vi "登录对话框.vi"() -> (1 "显示文件名":string, 2 "access out":T1)   [LabVIEW 2014]
uses:
  <vilib>/addons/database/Connection.llb/Conn ObjectReference.ctl
  <vilib>/addons/database/NI_Database_API.lvlib
panel:
  in  "Volume of rock sample(cm3)":string
  in  "Sectional area(cm2)":string
  in  "Irreducible water saturation(%)":string
  in  "Outlet pressure(MPa)":string
  in  "Inlet pressure(MPa)":string
  in  "Porosity(%)":string
  in  "Rock sample diameter(cm)":string
  in  "Injection water density(g/cm3)":string
  in  "Simulated oil density(g/cm3)":string
  in  "Air permeability(0.001um2)":string
  in  "Core depth(m)":string
  in  "Pore volume(cm3)":string
  in  "Length of rock sample(cm)":string
  in  "Injection water viscosity(mPa.S)":string
  in  "Simulated oil viscosity(mPa.S)":string
  in  "Experimental temperature(℃)":string
  in  "Lithological character":string
  in  "No.":string
  in  "Date of experiment":timestamp
  in  "Well number":string
  in  "Inspection item":string
  in  "取消按钮":bool
  in  "确定按钮":bool
  in  "Data store path":path
  in  "Document name":string
  # "Store path settings"
  # "Basic data"
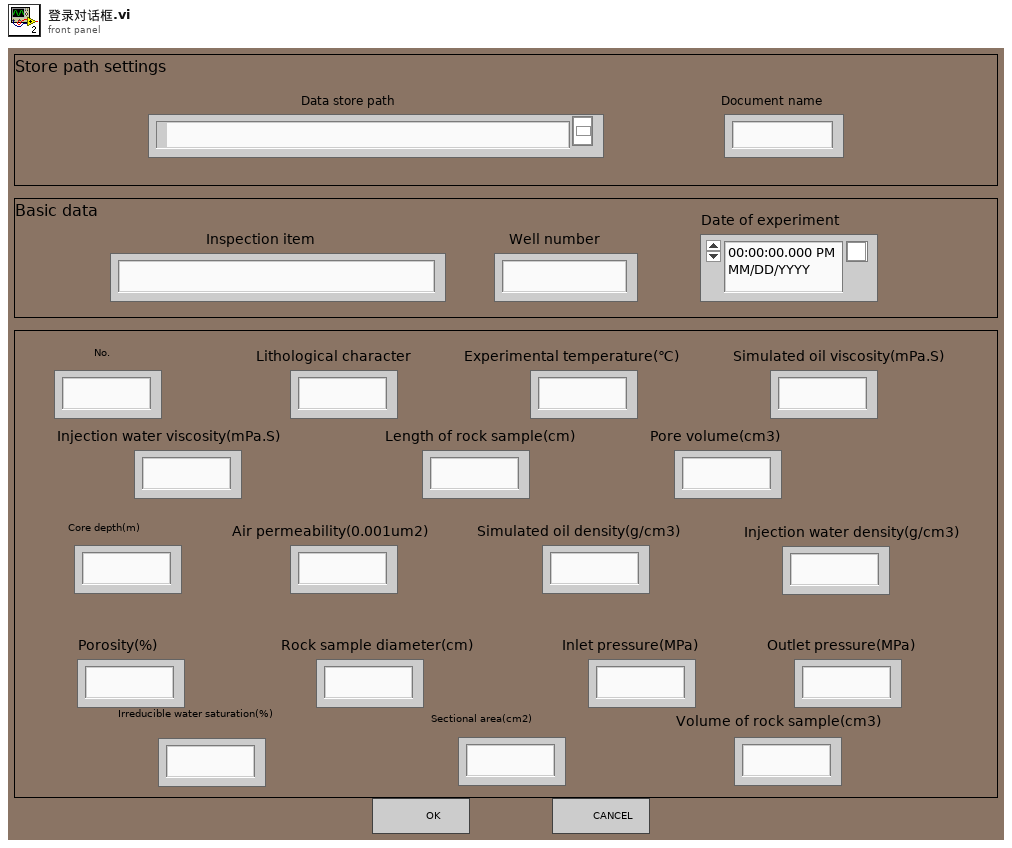
[diagram p1: front panel]
types:
  T1 = typedef "NI_Database_API.lvlib/Conn ObjectReference.ctl" = refnum<k1>
  T2 = cluster{"Inspection item":string, "Well number":string, "date/time string":string, "No.":string, "Lithological character":string, "Experimental temperature(℃)":string, "Simulated oil viscosity(mPa.S)":string, "Injection water viscosity(mPa.S) ":string, "Length of rock sample(cm)":string, "Pore volume(cm3) ":string, "Core depth(m)":string, "Air permeability(0.001um2)":string, "Simulated oil density(g/cm3)":string, "Injection water density(g/cm3)":string, "Porosity(%)":string, "Rock sample diameter(cm)":string, "Inlet pressure(MPa)":string, "Outlet pressure(MPa)":string, "Irreducible water saturation(%)":string, "Sectional area(cm2)":string, "Volume of rock sample(cm3)":string}
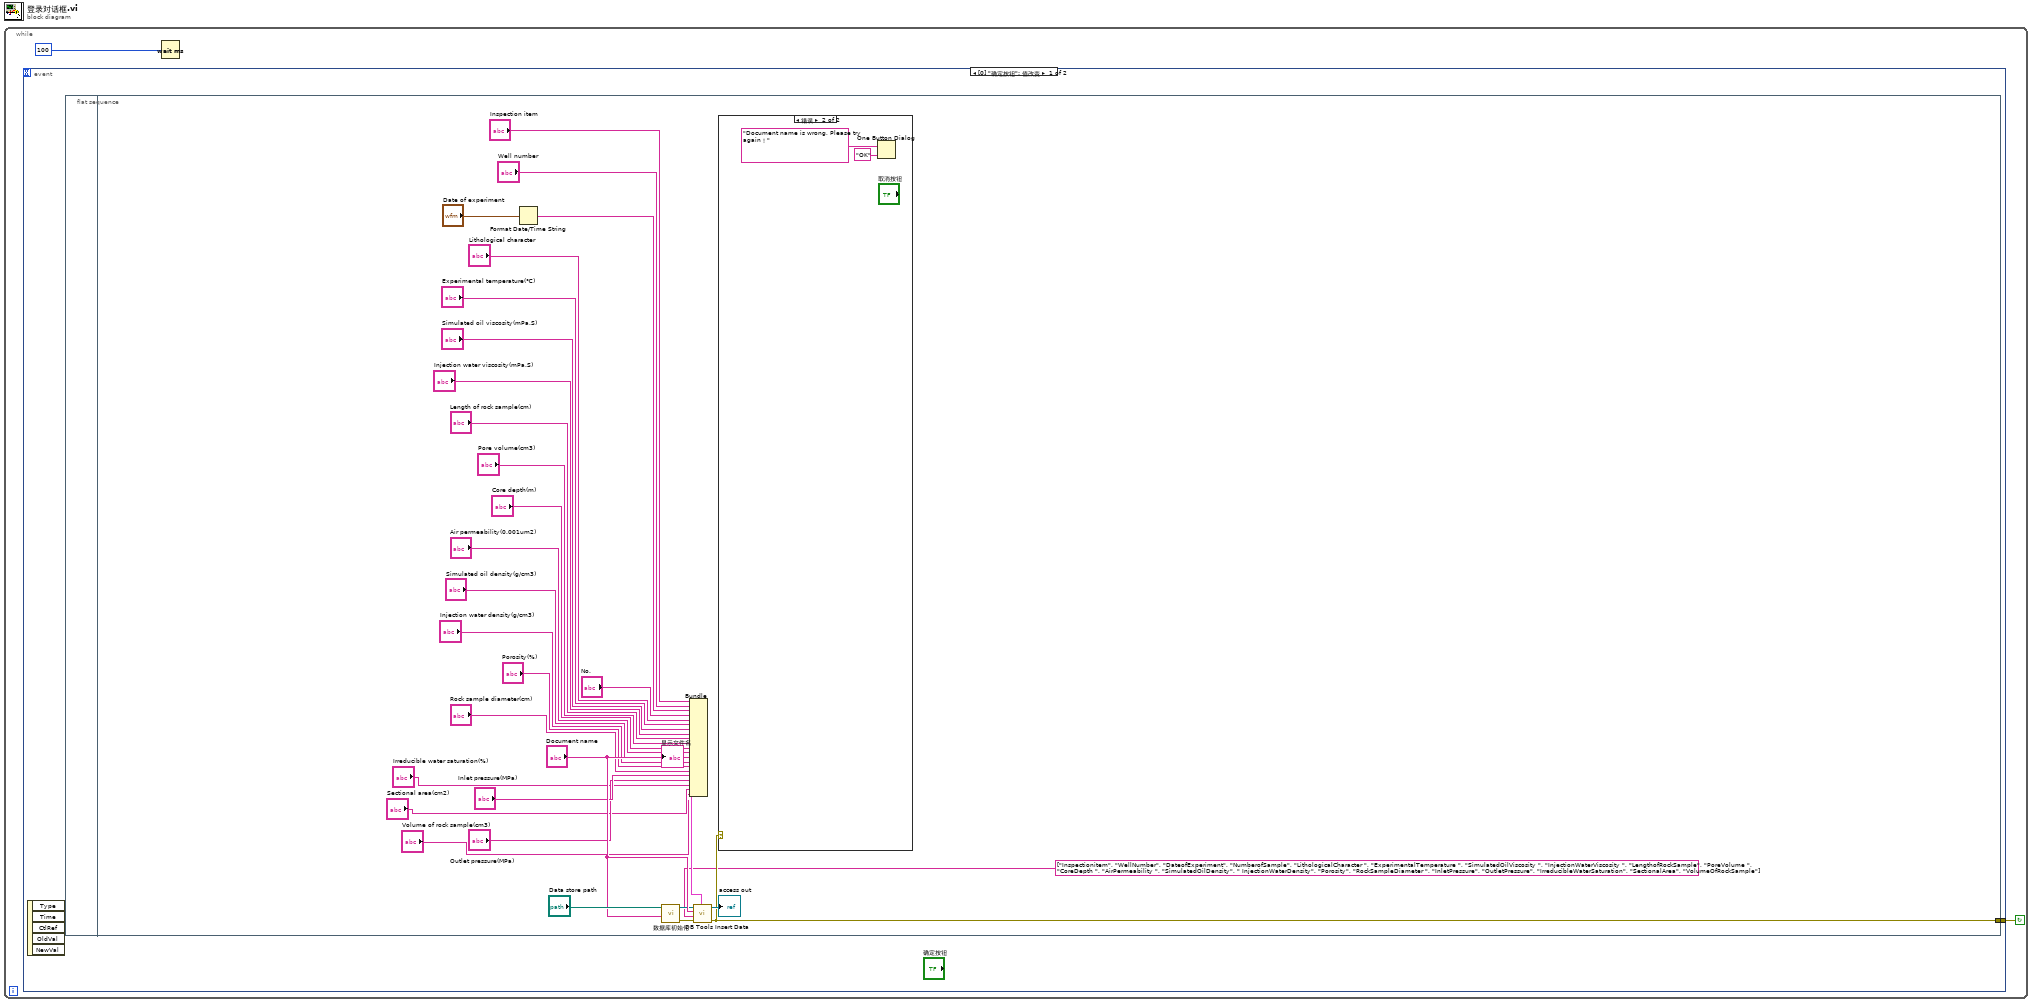
[diagram p0: block diagram]
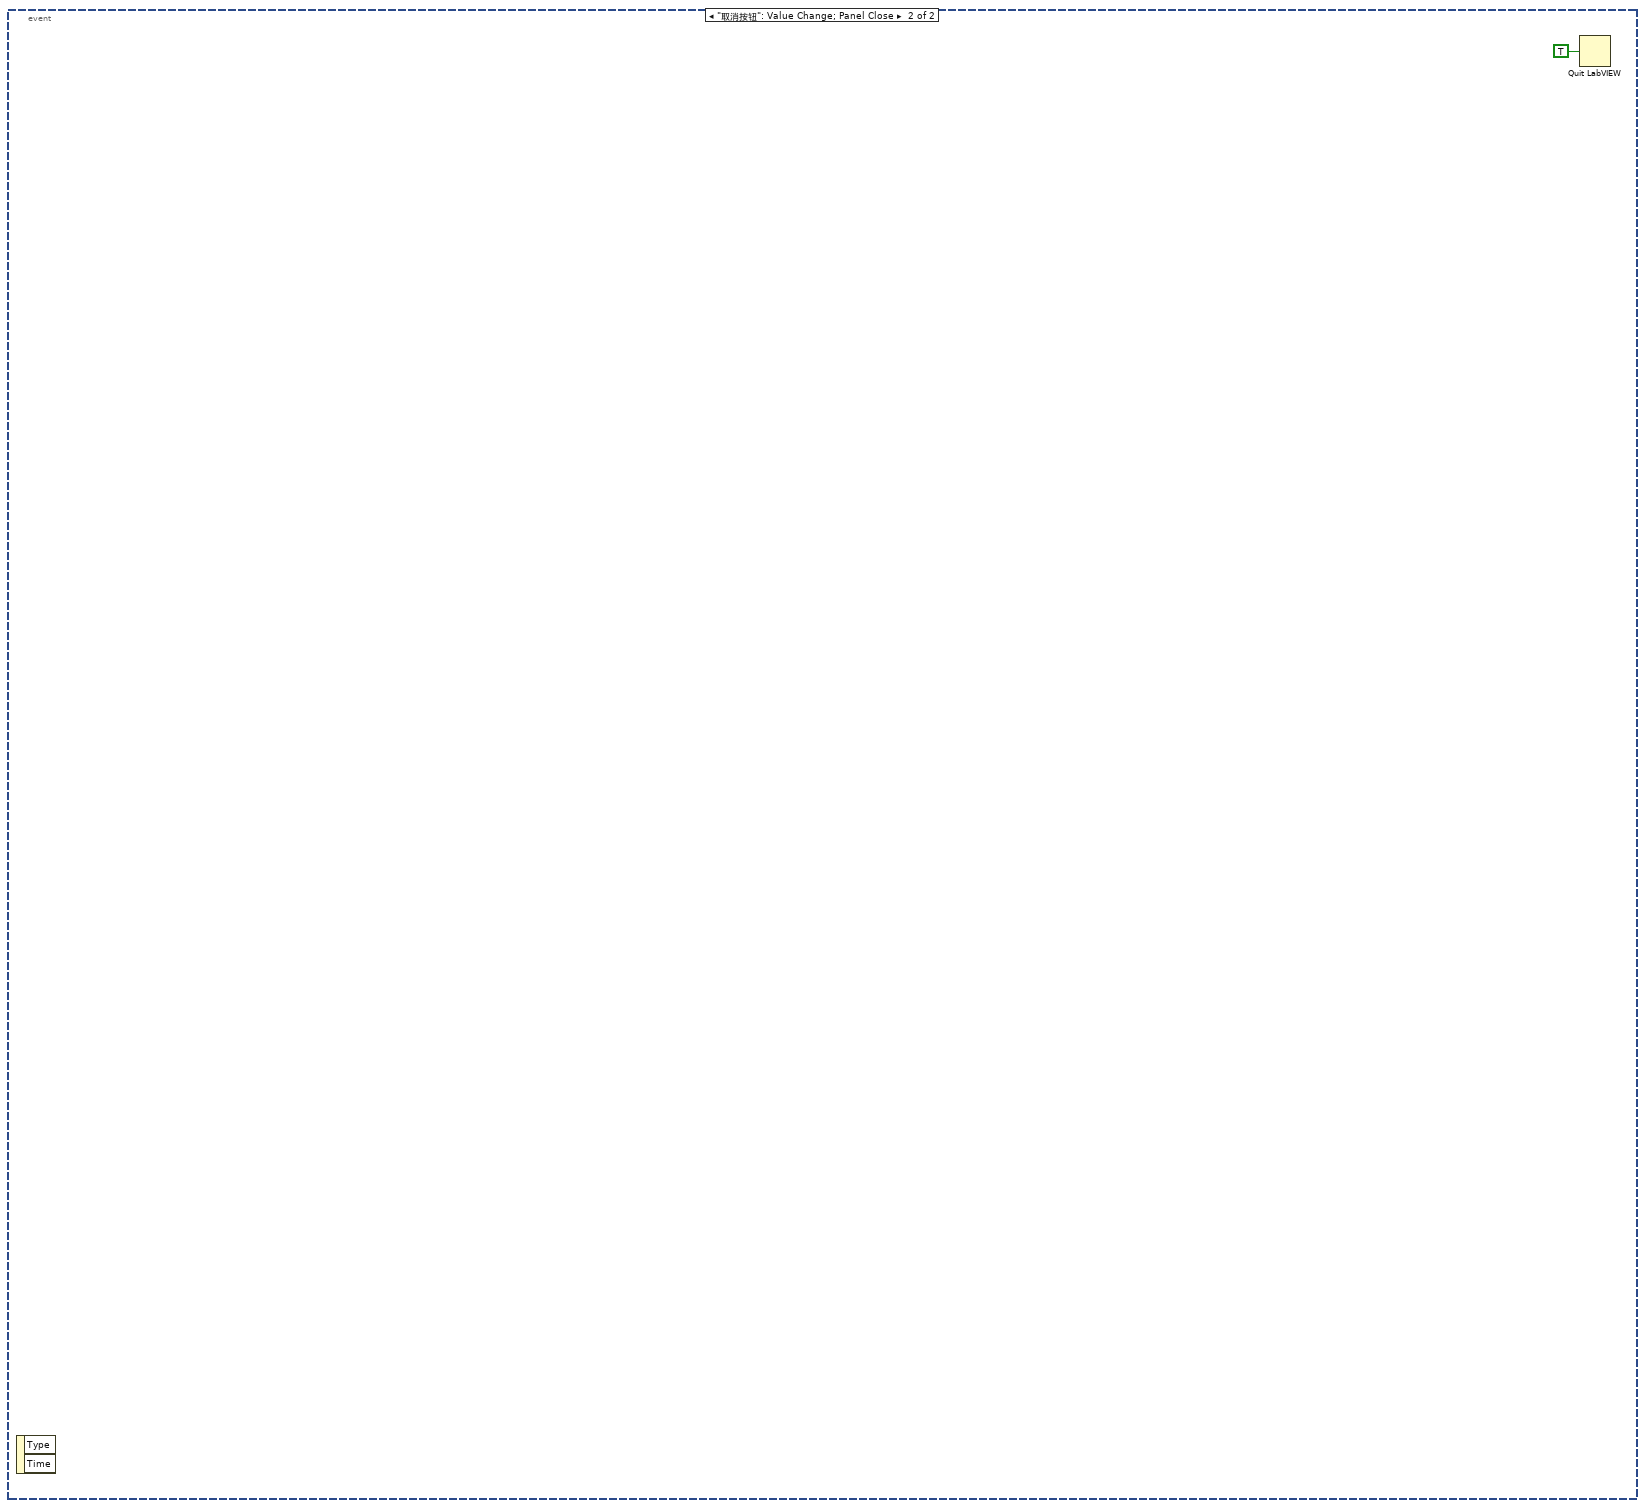
[diagram p3: hidden frame]
diagram:
  n1 = while {
    stop <- w2 continue-if-true
    n2 = event shown="[0] \"确定按钮\": 值改变" {
      selector: _ -> [_ _]
      dyn-events: _ -> [_ _]
      timeout: _ -> [_ _]
      tunnel: [w3 _] -> w2
      event "确定按钮": Value Change {
        n3 = event-data() -> ()  [unwired: 1 in, 5 out]
        n4 = flat-sequence {
          tunnel: [w28] -> w3
          frame #0 {
          }
          frame #1 {
            n5 = Format Date/Time String(seconds (now)="Date of experiment") -> (date/time string=w24:string)  [unwired: 2 in]
            n6 = call "数据库初始化.vi"("数据库文件名"="Document name", "数据保存路径"="Data store path") -> ("错误输出"=w30:errorcluster, "引用句柄输出"=w31:T1)  [unwired: 8 in]
            n7 = Bundle("Inspection item"="Inspection item", "Well number"="Well number", "date/time string"=w24, "No."="No.", "Lithological character"="Lithological character", "Experimental temperature(℃)"="Experimental temperature(℃)", "Simulated oil viscosity(mPa.S)"="Simulated oil viscosity(mPa.S)", "Injection water viscosity(mPa.S)"="Injection water viscosity(mPa.S)", "Length of rock sample(cm)"="Length of rock sample(cm)", "Pore volume(cm3)"="Pore volume(cm3)", "Core depth(m)"="Core depth(m)", "Air permeability(0.001um2)"="Air permeability(0.001um2)", "Simulated oil density(g/cm3)"="Simulated oil density(g/cm3)", "Injection water density(g/cm3)"="Injection water density(g/cm3)", "Porosity(%)"="Porosity(%)", "Rock sample diameter(cm)"="Rock sample diameter(cm)", "Inlet pressure(MPa)"="Inlet pressure(MPa)", "Outlet pressure(MPa)"="Outlet pressure(MPa)", "Irreducible water saturation(%)"="Irreducible water saturation(%)", "Sectional area(cm2)"="Sectional area(cm2)", "Volume of rock sample(cm3)"="Volume of rock sample(cm3)") -> (w10:T2)  [unwired: 1 in]
            n8 = call <vilib>:"DB Tools Insert Data.vi"("data"=w10, "error in (no error)"=w30, "columns"=string[] ["Inspectionitem", "WellNumber", "DateofExperiment", "NumberofSample", "LithologicalCharacter ", "ExperimentalTemperature ", "SimulatedOilViscosity ", "InjectionWaterViscosity ", "LengthofRockSample", "PoreVolume ", "CoreDepth ", "AirPermeability ", "SimulatedOilDensity", " InjectionWaterDensity", "Porosity", "RockSampleDiameter ", "InletPressure", "OutletPressure", "IrreducibleWaterSaturation", "SectionalArea", "VolumeOfRockSample"], "table"="Document name", "connection reference"=w31) -> ("error out"=w28:errorcluster, "connection reference out"=→"access out":T1)  [unwired: 5 in]
            n9 = case shown="错误" w28 {
              frame No Error {
              }
              frame Error {
                n10 = One Button Dialog(message="Document name is wrong, Please try again！" ("消息"), button name ("OK")="OK" ("按钮名称（“确定”）")) -> ()  [unwired: 1 out]
              }
            }
            "显示文件名" <- "Document name"
          }
        }
      }
      event "取消按钮": Value Change; Panel Close {
        n11 = event-data() -> ()  [unwired: 1 in, 2 out]
        n12 = Quit LabVIEW(quit? (T)=TRUE ("停止？(T)")) -> ()
      }
    }
    n13 = Wait (ms)(milliseconds to wait=u32 100 ("毫秒计时值")) -> ()  [unwired: 1 out]
  }
